vi "TwoBallAuto1.vi"() -> ()   [LabVIEW 2020]
uses:
  Global Variables/AutoTwoBalls.ctl
  Global Variables/Axes_N_Buttons.vi
  Global Variables/ActuatorsSensors.vi
panel:
  in  "Auto States":enum32{"PID Calibration", "Page 2"}(tab)
  out "Waveform Chart":dbl(graph)
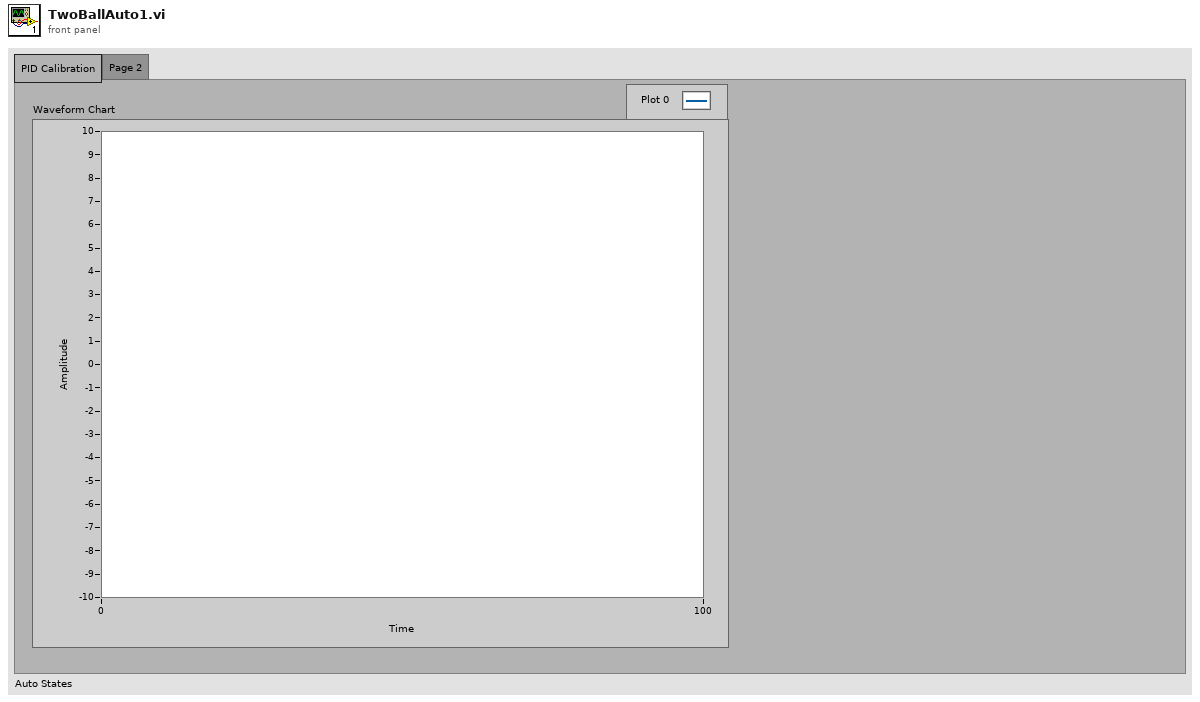
[diagram p1: front panel]
types:
  T1 = typedef "AutoTwoBalls.ctl" = enum16{"Start", "Collect Ball", "Delay 1", "Move to Tarmac", "Delay 2", "Align with the Hub", "Delay 3", "Backboard on the Wall", "Delay 4", "Prepare Shooter", "Shoot", "Reset"}
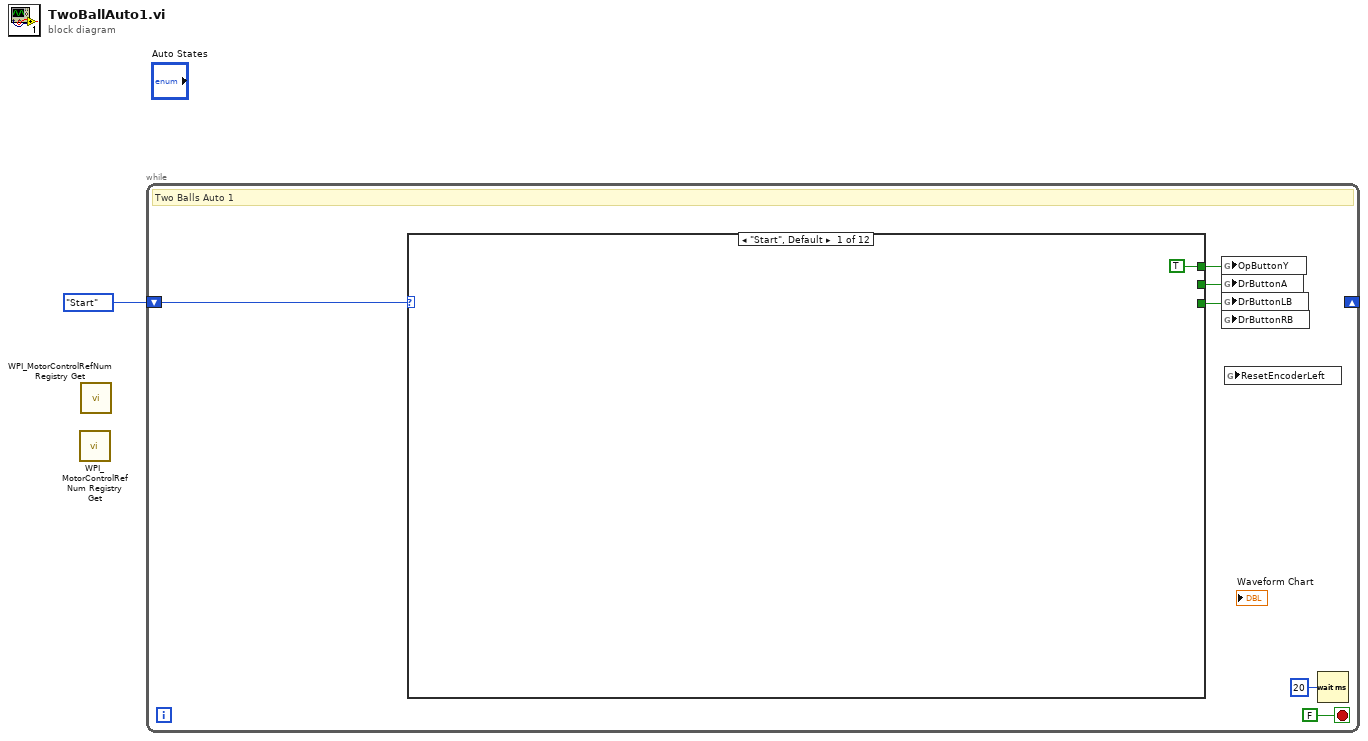
[diagram p0: block diagram]
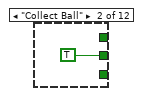
[diagram p2: hidden frame]
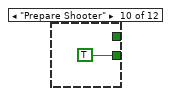
[diagram p10: hidden frame]
diagram:
  n1 = call <vilib>:"WPI_MotorControlRefNum Registry Get.vi"() -> ()  [unwired: 10 in, 2 out]
  n2 = call <vilib>:"WPI_MotorControlRefNum Registry Get.vi"() -> ()  [unwired: 10 in, 2 out]
  n3 = while {
    shift-right: _ -> [_]
    shift-left: AutoTwoBalls."Start" ("Enum") -> [w7]
    stop <- FALSE stop-if-true
    # "Two Balls Auto 1"
    n4 = case shown="\"Start\", Default" w7 {
      tunnel: [_ _ _ _ _ _ _ _ _ TRUE ("DrButtonLB") _ _] -> w4
      tunnel: [TRUE ("OpButtonY") _ _ _ _ _ _ _ _ _ _ _] -> w3
      tunnel: [_ TRUE ("OpButtonB") _ _ _ _ _ _ _ _ _ _] -> w2
      frame "Start", Default {
      }
      frame "Collect Ball" {
      }
      frame "Delay 1" {
      }
      frame "Move to Tarmac" {
      }
      frame "Delay 2" {
      }
      frame "Align with the Hub" {
      }
      frame "Delay 3" {
      }
      frame "Backboard on the Wall" {
      }
      frame "Delay 4" {
      }
      frame "Prepare Shooter" {
      }
      frame "Shoot" {
      }
      frame "Reset" {
      }
    }
    n5 = global write "Axes_N_Buttons.vi" "OpButtonY"(w3) -> ()
    n6 = global write "Axes_N_Buttons.vi" "DrButtonA"(w2) -> ()
    n7 = global write "Axes_N_Buttons.vi" "DrButtonLB"(w4) -> ()
    n8 = global read "Axes_N_Buttons.vi" "DrButtonRB"() -> ()  [unwired: 1 in]
    n9 = global read "ActuatorsSensors.vi" "ResetEncoderLeft"() -> ()  [unwired: 1 in]
    n10 = Wait (ms)(milliseconds to wait=u32 20) -> ()  [unwired: 1 out]
  }
